vi "DistanciaGoleiroBola.vi"(8 "Y bola":dbl format="%#_13g", 9 "X bola":dbl format="%#_13g", 10 "Y goleiro":dbl format="%#_13g", 11 "X goleiro":dbl format="%#_13g") -> (3 "Distância":dbl format="%#_13g")   [LabVIEW 2017]
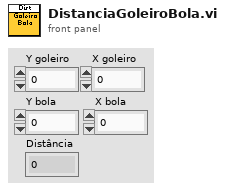
[diagram p1: front panel]
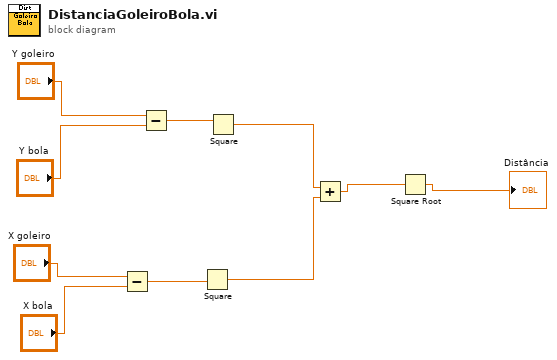
[diagram p0: block diagram]
diagram:
  n1 = Subtract(x="X goleiro", y="X bola") -> (x-y=w5:dbl)
  n2 = Subtract(x="Y goleiro", y="Y bola") -> (x-y=w6:dbl)
  n3 = Square(x=w5) -> (x^2=w3:dbl)
  n4 = Square(x=w6) -> (x^2=w4:dbl)
  n5 = Add(x=w4, y=w3) -> (x+y=w2:dbl)
  n6 = Square Root(x=w2) -> (sqrt(x)=→"Distância":dbl)
